vi "Launch GobangBoard.vi"() -> ()   [LabVIEW 2014, in "GoBang.lvlib"]
uses:
  GoBang.lvlib
  CS++GoBangClient.lvclass
  <vilib>/ActorFramework/Actor/Actor.lvclass
panel:
  out "error out":errorcluster
  in  "ini file":path
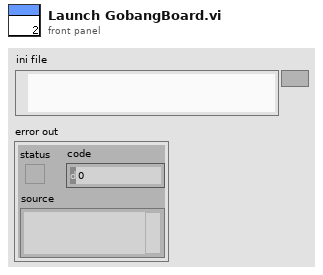
[diagram p1: front panel]
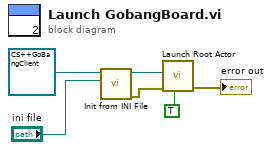
[diagram p0: block diagram]
diagram:
  n1 = call "Init from INI File.vi"("ini file"="ini file", "CS++GoBangClient in"=refnum<class "CS++GoBangClient.lvclass"> refnum ("GoBang.lvlib:CS++GoBangClient.lvclass")) -> ("error out"=w4:errorcluster, "CS++GoBangClient out"=w5:refnum<class "CS++GoBangClient.lvclass">)  [unwired: 8 in]
  n2 = call <vilib>:"Launch Root Actor.vi"("Open Actor Core front panel? (F)"=TRUE, "error in (no error)"=w4, "Actor"=w5) -> ("error out"=→"error out":errorcluster)  [unwired: 7 in, 1 out]
